vi "Initialize Front Panel.vi"(8 "error in (no error)":errorcluster, 11 "VerticalSlide In":refnum<class "PauseResumeButtons.lvclass">) -> (0 "error out":errorcluster, 3 "VerticalSlide Out":refnum<class "PauseResumeButtons.lvclass">)   [LabVIEW 2017, in "MVAExamples.lvlib" / "PauseResumeButtons.lvclass"]
doc: "<License>\nCopyright © 2017 Composed Systems, LLC | All rights reserved\nwww.composed.io\n\nAuthor: Ethan Stern <ethan.stern@composed.io>\n\nThis software is provided \"AS IS\" WITHOUT WARRANTIES, either express or implied, AND IS FOR EDUCATIONAL PURPOSES ONLY.\n</License>"
uses:
  PauseResumeButtons.lvclass
  PauseResumeButtons.lvclass/PauseResumeButtons.ctl
  Framework/IViewable/IViewable/IViewable.lvclass
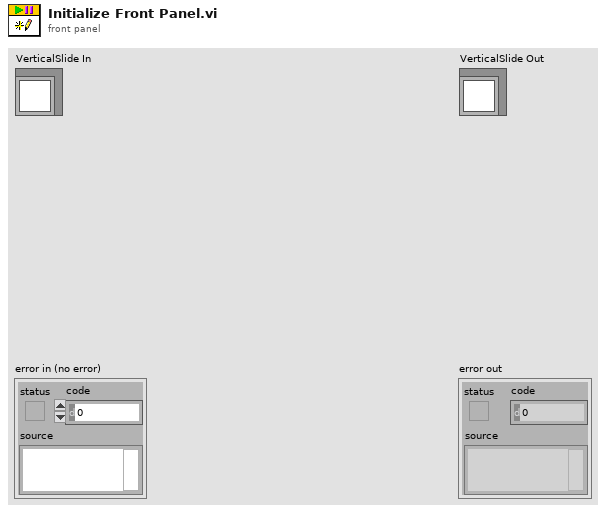
[diagram p1: front panel]
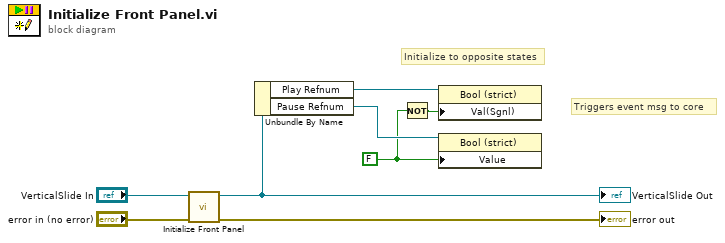
[diagram p0: block diagram]
diagram:
  w1 = FALSE ("Value")
  # "Triggers event msg to core"
  # "Initialize to opposite states"
  n1 = call-parent "Initialize Front Panel.vi"("error in (no error)"="error in (no error)", "IViewable in"="VerticalSlide In") -> ("error out"=→"error out":errorcluster, "IViewable out"=w5:refnum<class "PauseResumeButtons.lvclass">)  [unwired: 8 in]
  "VerticalSlide Out" <- w5
  n2 = Unbundle By Name(w5) -> ("Play Refnum"=w4:refnum<vi>, "Pause Refnum"=w3:refnum<vi>)
  n3 = Not(x=w1) -> (.not. x?=w2:bool)
  n4 = property class="Bool (strict)"(reference=w4, "Val(Sgnl)"=w2) -> ()  [unwired: 1 in, 2 out]
  n5 = property class="Bool (strict)"(reference=w3, "Value"=w1) -> ()  [unwired: 1 in, 2 out]
